vi "niFPGA Threshold Crossing with I.C. (I16).vi"(5 "reset":bool, 6 "low ref level":i16, 7 "high ref level":i16, 8 "state in":T1={"level"=[FALSE, FALSE, FALSE, FALSE, FALSE, FALSE], "rising?"=FALSE, "hi hyst met?"=FALSE, "lo hyst met?"=FALSE, "gt threshold"=FALSE, "lt threshold"=FALSE}, 9 "direction":u8(ring) items=["falling", "rising"], 10 "threshold":i16, 11 "input data":i16) -> (0 "state out":T1, 3 "crossing":bool)   [LabVIEW 2017]
uses:
  <vilib>/rvi/Analysis/utilities/niFPGA Threshold Crossing State.ctl
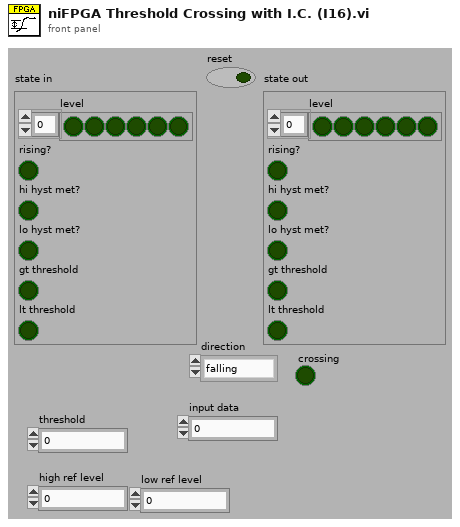
[diagram p1: front panel]
types:
  T1 = typedef "niFPGA Threshold Crossing State.ctl" = cluster{"level":bool[], "rising?":bool, "hi hyst met?":bool, "lo hyst met?":bool, "gt threshold":bool, "lt threshold":bool}
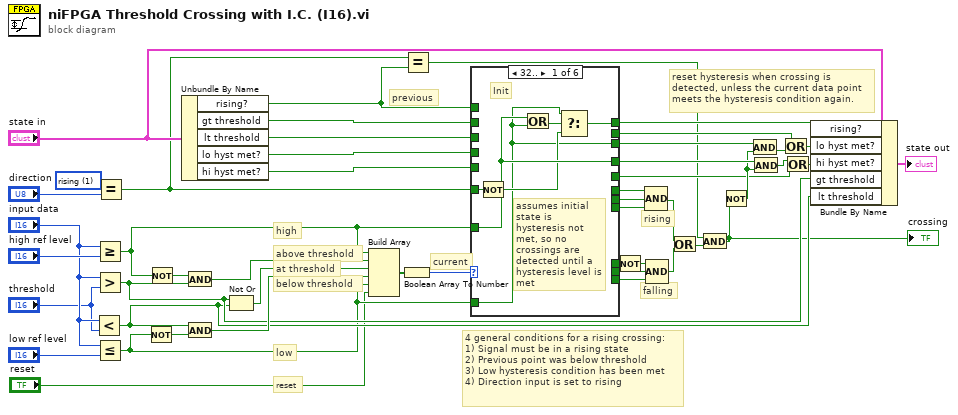
[diagram p0: block diagram]
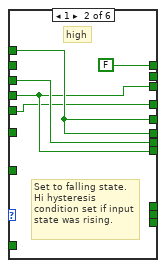
[diagram p2: hidden frame]
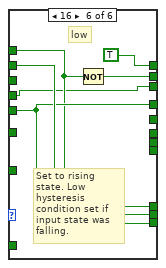
[diagram p6: hidden frame]
diagram:
  w25 = u8 1 items=["falling", "rising"] ("direction")
  # "reset"
  # "low"
  # "below threshold"
  # "at threshold"
  # "above threshold"
  # "high"
  # "rising"
  # "falling"
  # "reset hysteresis when crossing is detected, unless the current data point meets the hysteresis condition again."
  # "4 general conditions for a rising crossing:\n1) Signal must be in a rising state\n2) Previous point was below threshold\n3) Low hysteresis condition has been met\n4) Direction input is set to rising"
  # "current"
  # "previous"
  n1 = Less?(x="input data", y="threshold") -> (x < y?=w30:bool)
  n2 = Greater Or Equal?(x="input data", y="high ref level") -> (x >= y?=w26:bool)
  n3 = Greater?(x="input data", y="threshold") -> (0:w31:bool)
  n4 = Less Or Equal?(x="input data", y="low ref level") -> (x <= y?=w5:bool)
  n5 = Equal?(x=w25, y="direction") -> (x = y?=w1:bool)
  n6 = Not(x=w5) -> (.not. x?=w43:bool)
  n7 = Not(x=w26) -> (.not. x?=w44:bool)
  n8 = Unbundle By Name("state in") -> ("rising?"=w27:bool, "gt threshold"=w34:bool, "lt threshold"=w33:bool, "lo hyst met?"=w28:bool, "hi hyst met?"=w32:bool)
  n9 = And(x=w44, y=w31) -> (x .and. y?=w42:bool)
  n10 = And(x=w30, y=w43) -> (x .and. y?=w39:bool)
  n11 = Not Or(1:w30, 2:w31) -> (0:w41:bool)
  n12 = Build Array(w26, w42, w41, w39, w5, "reset") -> (w35:bool[])
  n13 = Boolean Array To Number(Boolean array=w35) -> (number=w40:u8)
  n14 = Equal?(x=w1, y=w27) -> (x = y?=w2:bool)
  n15 = case shown="32.." w40 {
    tunnel: [_ _ _ w68 w71 w75] -> w12
    tunnel: [w49 FALSE w62 w68 w71 TRUE] -> w36
    tunnel: w27 -> [_ w57 w62 w68 w71 w75]
    tunnel: w34 -> [_ _ _ w65 w70 w77]
    tunnel: w33 -> [_ w58 w61 w64 _ _]
    tunnel: w32 -> [_ w55 w63 w66 w69 w76]
    tunnel: [w53 w55 w63 w66 w69 w76] -> w24
    tunnel: [w50 w56 w60 w67 w72 w73] -> w23
    tunnel: w28 -> [_ w56 w60 w67 w72 w73]
    tunnel: w5 -> [w50 _ _ _ _ _]
    tunnel: w26 -> [w53 _ _ _ _ _]
    tunnel: [_ _ _ _ _ w74] -> w18
    tunnel: [_ w57 _ _ _ _] -> w16
    tunnel: [_ w57 w62 w68 _ _] -> w11
    tunnel: [_ w58 w61 w67 _ _] -> w10
    tunnel: [_ w56 w60 w64 _ _] -> w9
    tunnel: [_ _ _ w66 w70 w77] -> w8
    tunnel: [_ _ _ w65 w69 w76] -> w7
    tunnel: w1 -> [w52 _ _ _ _ _]
    frame 32.. {
      # "assumes initial state is hysteresis not met, so no crossings are detected until a hysteresis level is met"
      # "Init"
      n16 = Not(x=w52) -> (.not. x?=w51:bool)
      n17 = Or(x=w53, y=w50) -> (x .or. y?=w54:bool)
      n18 = Select(t=w50, s=w54, f=w51) -> (s? t:f=w49:bool)
    }
    frame 1 {
      # "Set to falling state. Hi hysteresis condition set if input state was rising."
      # "high"
    }
    frame 2 {
      # "above threshold"
    }
    frame 4, Default {
      # "falling crossing"
      # "rising crossing"
      # "== threshold"
    }
    frame 8 {
      # "below threshold"
    }
    frame 16 {
      # "Set to rising state. Low hysteresis condition set if input state was falling."
      # "low"
      n19 = Not(x=w75) -> (.not. x?=w74:bool)
    }
  }
  n20 = Not(x=w12) -> (.not. x?=w6:bool)
  n21 = Compound Arithmetic op=AND(w11, w10, w9) -> (w14:bool)
  n22 = Compound Arithmetic op=AND(w6, w8, w7) -> (w15:bool)
  n23 = Or(x=w14, y=w15) -> (x .or. y?=w13:bool)
  n24 = And(x=w2, y=w13) -> (x .and. y?=w3:bool)
  "crossing" <- w3
  n25 = Not(x=w3) -> (.not. x?=w17:bool)
  n26 = And(x=w23, y=w17) -> (x .and. y?=w22:bool)
  n27 = And(x=w24, y=w17) -> (x .and. y?=w21:bool)
  n28 = Or(x=w18, y=w22) -> (x .or. y?=w19:bool)
  n29 = Or(x=w21, y=w16) -> (x .or. y?=w20:bool)
  n30 = Bundle By Name(cluster="state in", "rising?"=w36, "lo hyst met?"=w19, "hi hyst met?"=w20, "gt threshold"=w31, "lt threshold"=w30) -> (→"state out":T1)
